vi "IMS Stepper Init.vi"(4 "error in (no error)":errorcluster, 5 "Baud Rate":u32=9600, 6 "Motor Number":u32=1 min=1 max=255 step=1, 7 "Instrument Address":refnum<visa-resource-name>) -> (0 "error out":errorcluster, 2 "Response":string, 3 "dup VISA Resource Name":refnum<visa-resource-name>)   [LabVIEW 2020]
uses:
  Serial Support VISA.llb/Serial Actions.ctl
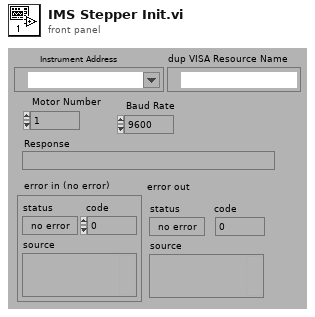
[diagram p1: front panel]
types:
  T1 = cluster{"flow control":enum16{"None", "XON/XOFF", "RTS/CTS"}, "baud rate":u32, "data bits":u16, "Stop Bits":u16, "parity (0:none)":enum16{"None", "Odd", "Even", "Mark", "Space"}, "Transmit Buffer Size":u32, "Receive Buffer Size":u32}
  T2 = typedef "Serial Actions.ctl" = enum16{"Init", "Break", "Clear Buffer", "Write", "Read", "N Bytes", "Lock", "Unlock", "Close"}
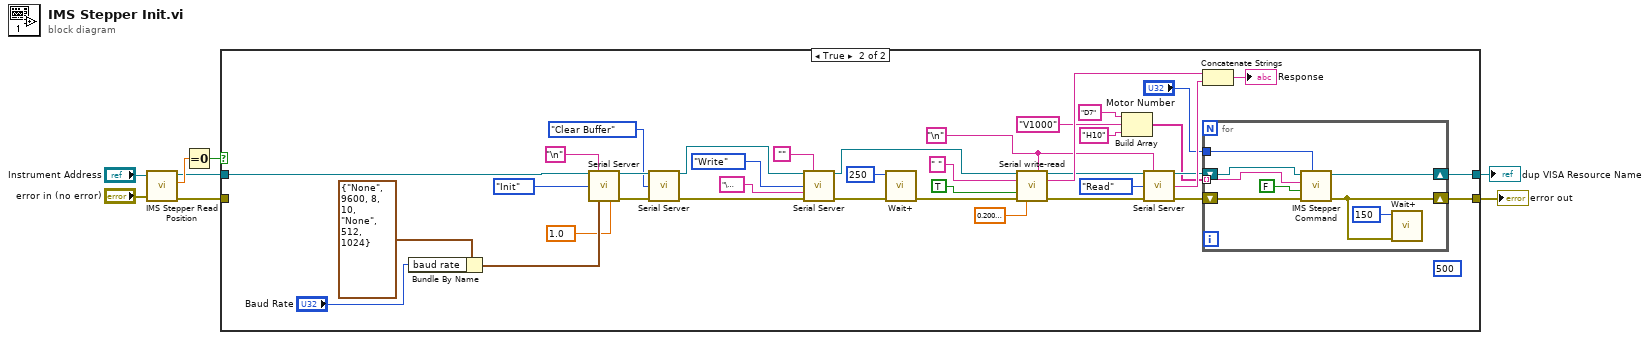
[diagram p0: block diagram]
diagram:
  n1 = call "IMS Stepper Read Position.vi"("Instrument Address"="Instrument Address", "error in (no error)"="error in (no error)") -> ("Instrument Address Out"=w2:refnum<visa-resource-name>, "Response"=w8:dbl, "error out"=w7:errorcluster)  [unwired: 2 in]
  n2 = Equal To 0?(x=w8) -> (x = 0?=w3:bool)
  n3 = case shown="True" w3 {
    tunnel: w7 -> [w10 _]
    tunnel: w2 -> [w9 w14]
    tunnel: [w10 w13] -> w4
    tunnel: [w9 w11] -> w1
    frame False {
    }
    frame True {
      w31 = "\n" ("EOT Chars (cr/lf)")
      (unwired) u32 500 ("Max Char to Read")
      n4 = Bundle By Name(cluster=T1 {"flow control"=enum."None", "baud rate"=9600, "data bits"=8, "Stop Bits"=10, "parity (0:none)"=enum."None", "Transmit Buffer Size"=512, "Receive Buffer Size"=1024} ("Port Parameters"), "baud rate"="Baud Rate") -> (w24:T1)
      n5 = call "Serial Server.vi"("VISA Resource Name"=w14, "EOT Chars (cr/lf)"="\n", "Action"=Serial_Actions."Init", "Port Parameters"=w24, "Timeout Limit(sec)"=1.0 ("Timeout Limit")) -> ("dup VISA Resource Name"=w23:refnum<visa-resource-name>, "error out"=w20:errorcluster)  [unwired: 6 in, 3 out]
      n6 = call "Serial Server.vi"("VISA Resource Name"=w23, "Action"=Serial_Actions."Clear Buffer", "error in (no error)"=w20) -> ("dup VISA Resource Name"=w47:refnum<visa-resource-name>, "error out"=w46:errorcluster)  [unwired: 8 in, 3 out]
      n7 = call "Serial Server.vi"("VISA Resource Name"=w47, "EOT Chars (cr/lf)"="", "Action"=Serial_Actions."Write", "String To Send"="\u0003" ("Command"), "error in (no error)"=w46) -> ("dup VISA Resource Name"=w48:refnum<visa-resource-name>, "error out"=w41:errorcluster)  [unwired: 6 in, 3 out]
      n8 = call "Wait+.vi"("Error In"=w41, "milliseconds to wait"=u32 250) -> ("Error Out"=w45:errorcluster)  [unwired: 4 in, 1 out]
      n9 = call "Serial write-read.vi"("VISA Resource Name"=w48, "EOT Chars (cr/lf)"=w31, "String To Send"=" " ("Command"), "Clear Buffer?"=TRUE, "error in (no error)"=w45, "Timeout Limit"=sgl 0.2) -> ("dup VISA Resource Name"=w35:refnum<visa-resource-name>, "Serial Read"=w37:string, "error out"=w36:errorcluster)  [unwired: 4 in, 3 out]
      n10 = Build Array("D7", "V1000", "H10") -> (w16:string[])
      n11 = call "Serial Server.vi"("VISA Resource Name"=w35, "EOT Chars (cr/lf)"=w31, "Action"=Serial_Actions."Read", "error in (no error)"=w36) -> ("dup VISA Resource Name"=w33:refnum<visa-resource-name>, "Serial Read"=w39:string, "error out"=w32:errorcluster)  [unwired: 7 in, 2 out]
      n12 = Concatenate Strings(w37, w39) -> (→"Response":string)
      n13 = for {
        shift-right: [w51] -> w13
        shift-left: w32 -> [w52]
        tunnel: w16 -> [w55] mode=indexing
        tunnel: "Motor Number" -> [w54]
        shift-right: [w49] -> w11
        shift-left: w33 -> [w53]
        n14 = call "IMS Stepper Command.vi"("Motor Number"=w54, "error in (no error)"=w52, "Mode"=FALSE, "Command"=w55, "Instrument Address"=w53) -> ("error out"=w51:errorcluster, "Instrument Address Out"=w49:refnum<visa-resource-name>)  [unwired: 1 in, 2 out]
        n15 = call "Wait+.vi"("Error In"=w51, "milliseconds to wait"=u32 150) -> ()  [unwired: 4 in, 2 out]
      }
    }
  }
  "error out" <- w4
  "dup VISA Resource Name" <- w1
